vi "Add Network Chassis.vi"(0 "session in":refnum<k21>, 1 "username":string, 2 "password":string, 5 "chassis IP address/hostname":string, 11 "error in (no error)":errorcluster, 12 "connect timeout (60 sec)":dbl=60.0) -> (4 "session out":refnum<k21>, 6 "chassis out":refnum<k21>, 15 "error out":errorcluster)   [LabVIEW 2020, in "SLSC.lvlib"]
doc: "Adds the specified network chassis to the local configuration file. This VI connects to the specified network chassis, downloads information about the chassis and its modules, and adds the chassis and modules to the local configuration file. If the chassis has already been added, calling this function again refreshes the modules."
uses:
  <vilib>/SLSC/SLSC.lvlib
  nislsclvapi.dll
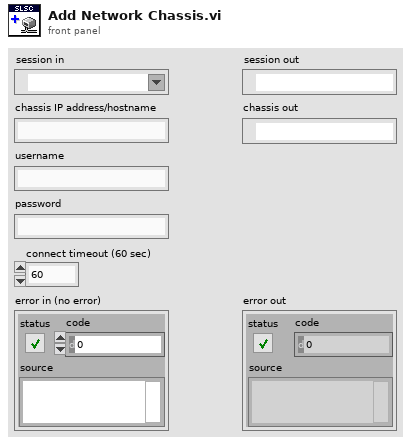
[diagram p1: front panel]
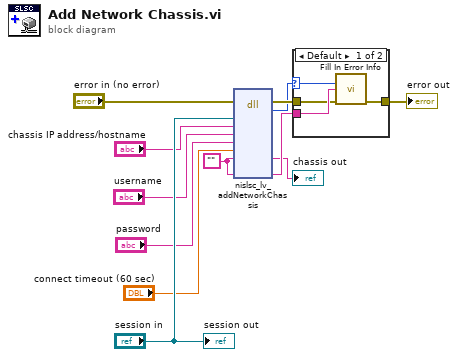
[diagram p0: block diagram]
diagram:
  w2 = ""
  n1 = dll-call lib="nislsclvapi.*" fn="nislsc_lv_addNetworkChassis"(error in="error in (no error)", "session"="session in", "address"="chassis IP address/hostname", "username"="username", "password"="password", "connectTimeout"="connect timeout (60 sec)", "chassis"=w2, "extendedErrorInfo"=w2) -> (error out=w9:errorcluster, "return type"=w8:i32, "chassis"=→"chassis out":string, "extendedErrorInfo"=w10:string)  [unwired: 9 in, 1 out]
  n2 = case shown="Default" w8 {
    selector: w8 -> [w16 _]
    tunnel: w10 -> [w15 _]
    tunnel: w9 -> [w14 w17]
    tunnel: [w13 w17] -> w7
    frame Default {
      n3 = call <vilib>:"Fill In Error Info.vi"("status code"=w16, "extended error info"=w15, "error in"=w14) -> ("error out"=w13:errorcluster)  [unwired: 12 in]
    }
    frame 0 {
    }
  }
  "error out" <- w7
  "session out" <- "session in"
